vi "CAD@LoadToolModel__Parameter.vi"(1 "ParamterIn":string) -> (0 "ParamterOut":string)   [LabVIEW 2020]
uses:
  MainFrame/Global.vi
panel:
  in  "PartName":string(combo)
  in  "Confirm":bool
  # "CAD@LoadToolModel $File.tool"
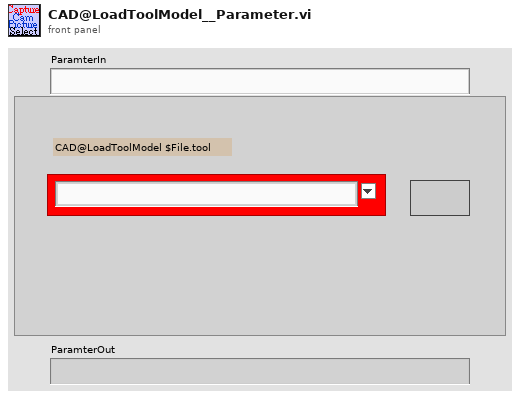
[diagram p1: front panel]
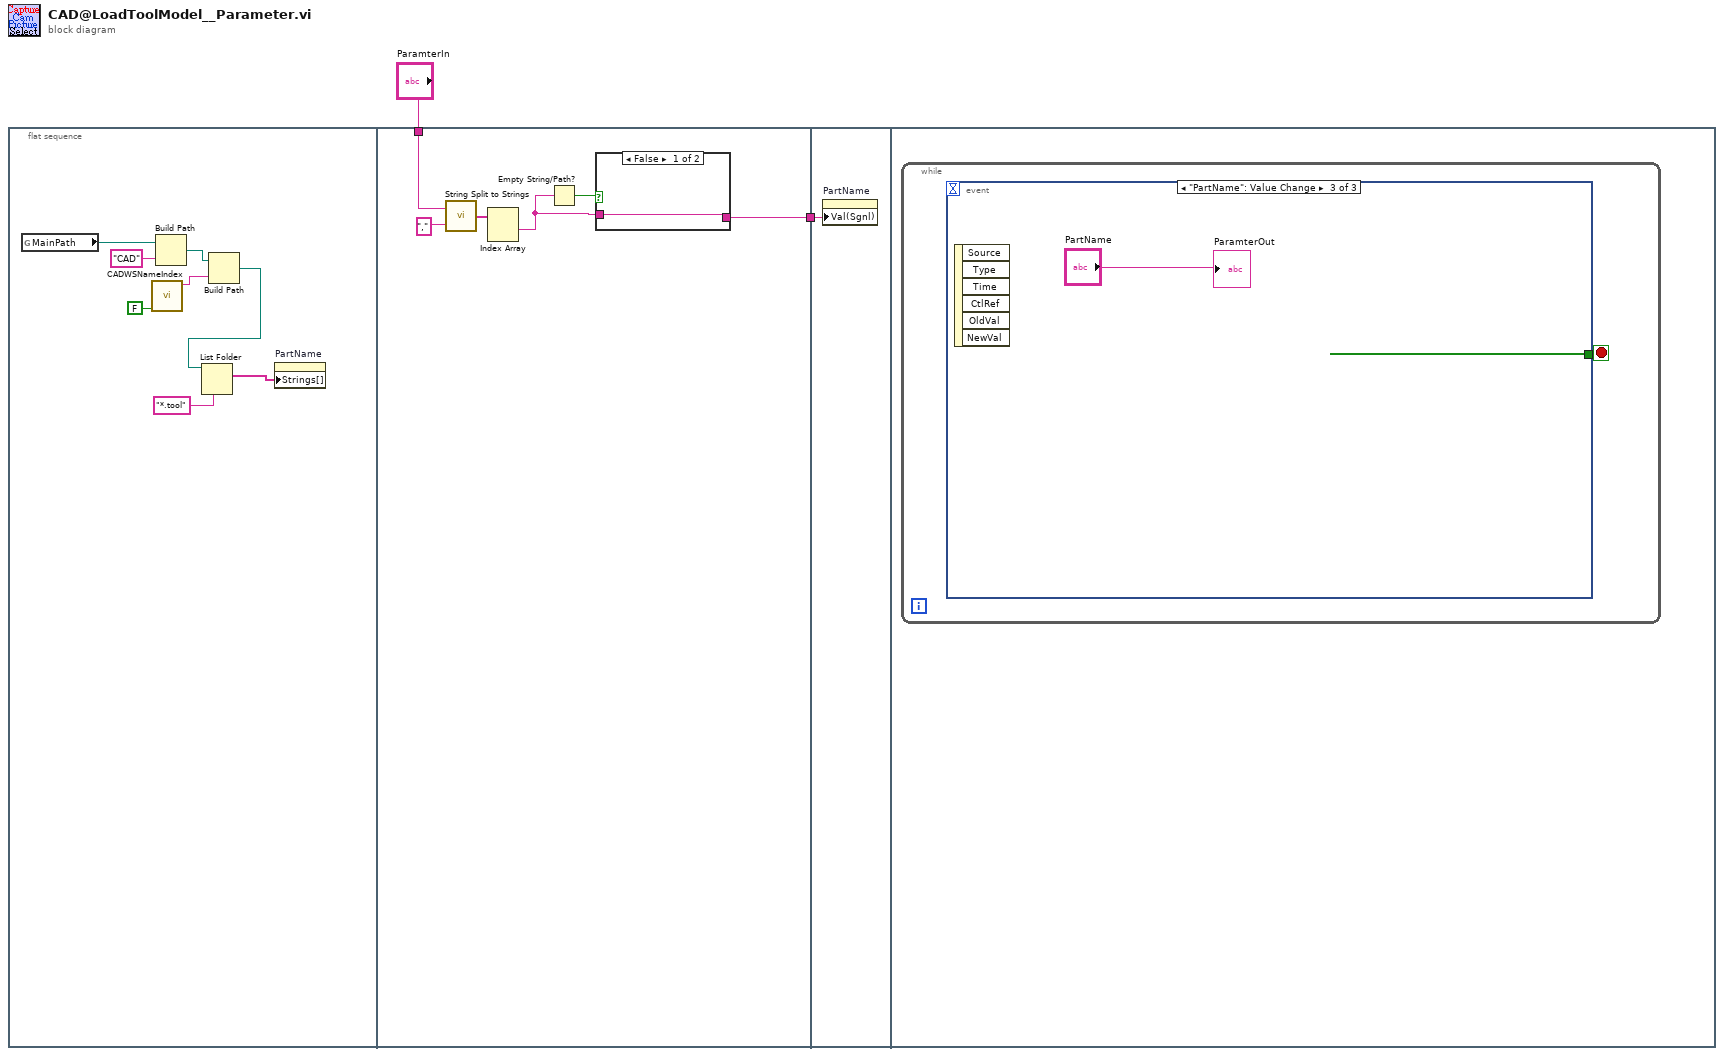
[diagram p0: block diagram]
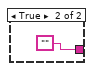
[diagram p2: hidden frame]
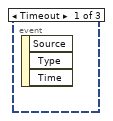
[diagram p3: hidden frame]
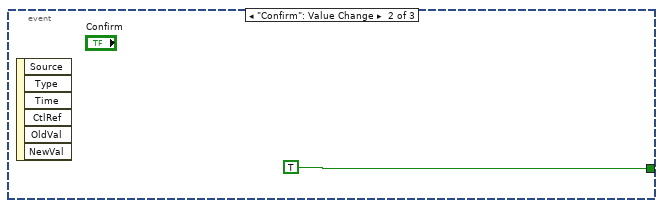
[diagram p4: hidden frame]
diagram:
  n1 = flat-sequence {
    tunnel: "ParamterIn" -> [w14]
    tunnel: [w12] -> w1
    tunnel: w1 -> [w19]
    frame #0 {
      n2 = global read "Global.vi" "MainPath"() -> (w10:path)
      n3 = call "CADWSNameIndex.vi"("Set"=FALSE) -> ("WorkSpaceOut"=w4:string)  [unwired: 10 in]
      n4 = Build Path(base path=w10, name or relative path="CAD") -> (appended path=w5:path)
      n5 = Build Path(base path=w5, name or relative path=w4) -> (appended path=w3:path)
      n6 = List Folder(path=w3, pattern="*.tool") -> (filenames=w7:string[])  [unwired: 2 in, 3 out]
      n7 = property on="PartName" class="CmbBox"("Strings[]"=w7) -> ()  [unwired: 2 in, 2 out]
    }
    frame #1 {
      n8 = call "String Split to Strings.vi"("search string/char (-)"=",", "String"=w14) -> ("Array"=w16:string[])
      n9 = Index Array(array=w16) -> (element #1=w11:string)  [unwired: 2 in, 1 out]
      n10 = Empty String/Path?(string/path=w11) -> (empty?=w13:bool)
      n11 = case shown="False" w13 {
        tunnel: [w17 ""] -> w12
        tunnel: w11 -> [w17 _]
        frame False {
        }
        frame True {
        }
      }
    }
    frame #2 {
      n12 = property on="PartName" class="CmbBox"("Val(Sgnl)"=w19) -> ()  [unwired: 2 in, 2 out]
    }
    frame #3 {
      n13 = while {
        stop <- w20 stop-if-true
        n14 = event shown="[2] \"PartName\": Value Change" {
          selector: _ -> [_ _ _]
          dyn-events: _ -> [_ _ _]
          timeout: _ -> [_ _ _]
          tunnel: [_ TRUE _] -> w20
          event Timeout {
            n15 = event-data() -> ()  [unwired: 1 in, 3 out]
          }
          event "Confirm": Value Change {
            n16 = event-data() -> ()  [unwired: 1 in, 6 out]
          }
          event "PartName": Value Change {
            n17 = event-data() -> ()  [unwired: 1 in, 6 out]
            "ParamterOut" <- "PartName"
          }
        }
      }
    }
  }
